vi "UpdateCaliperToCoorResultTable.vi"(7 "Type":enum16{"TagName", "Value"}(ring), 8 "error in (no error)":errorcluster, 10 "ProjectName":string, 11 "MCListbox Refnum":refnum<vi>) -> (0 "error out":errorcluster, 3 "CaliperResultNames":string[](array[string]))   [LabVIEW 2019]
uses:
  Controls/Caliper_Entry_FGV_Action.ctl
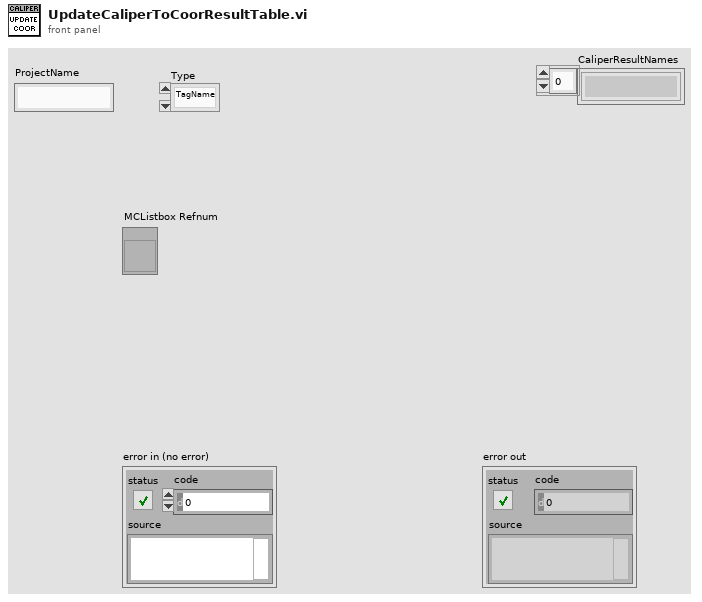
[diagram p1: front panel]
types:
  T1 = typedef "Caliper_Entry_FGV_Action.ctl" = enum16{"Init", "Close", "Add", "Delete", "ReplaceAll", "ReadAll"}
  T2 = typedef "CaliperDataEntry.ctl" = cluster{"CaliperType":T3, "Points":T4[], "Result":T6, "StepName":string}
  T3 = typedef "CaliperType.ctl" = u32
  T4 = typedef "SelectionListEntry.ctl" = cluster{"Type":T5, "Index":i32}
  T5 = typedef "SelectionListEntryPointType.ctl" = enum16{"AnalysisResult", "CaliperResult"}
  T6 = typedef "CaliperResult.ctl" = cluster{"PointInclude?":bool, "Num_Of_Pts":u8, "Position.X":dbl, "Position.Y":dbl, "Angle":dbl, "Distance":dbl, "Area":dbl, "Radius_MAX":dbl, "Radius2_min":dbl, "Dev_Residual":dbl, "P2.X":dbl, "P2.Y":dbl, "StepName":string, "Point ID":u8, "StepError?":bool, "ResultDiff?":bool}
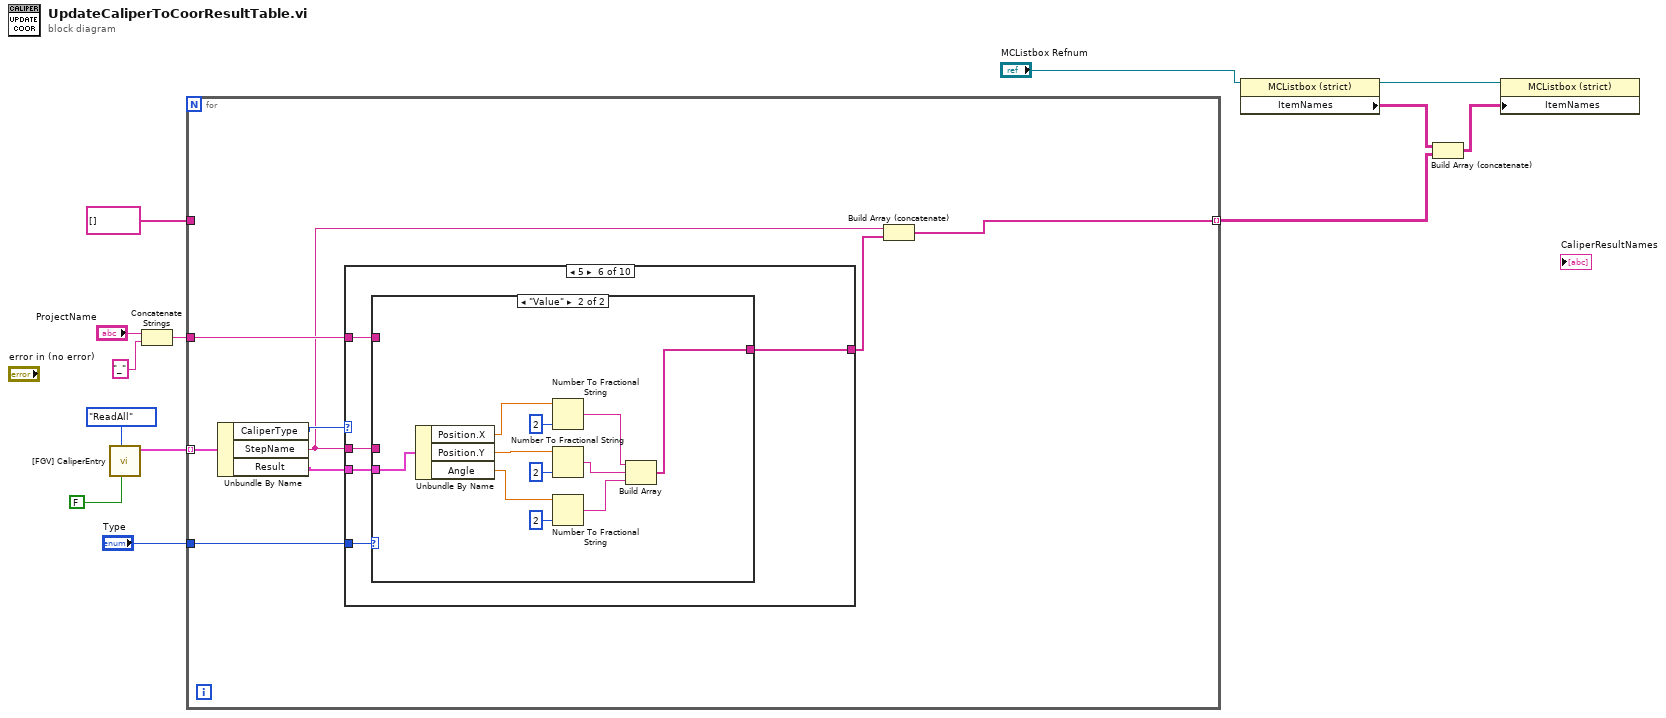
[diagram p0: block diagram]
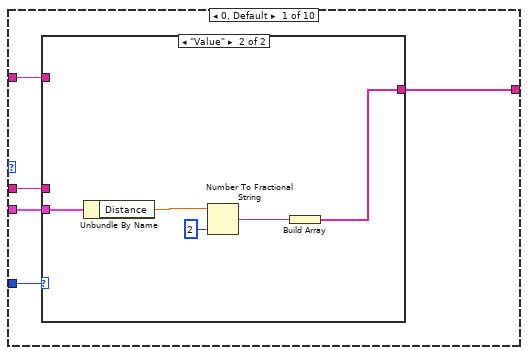
[diagram p2: hidden frame]
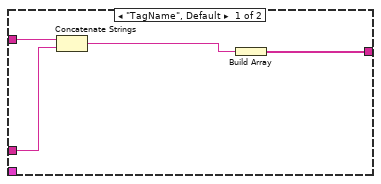
[diagram p3: hidden frame]
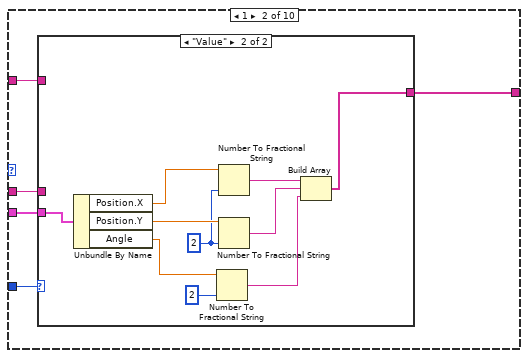
[diagram p4: hidden frame]
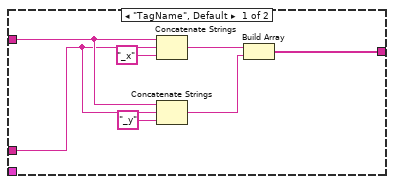
[diagram p5: hidden frame]
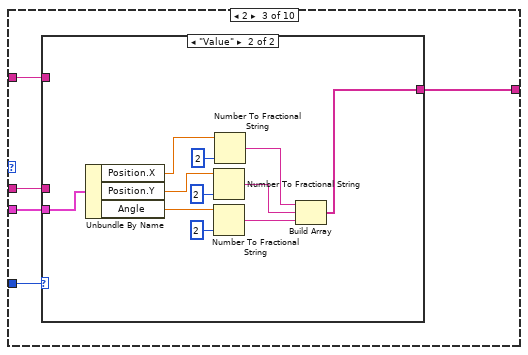
[diagram p6: hidden frame]
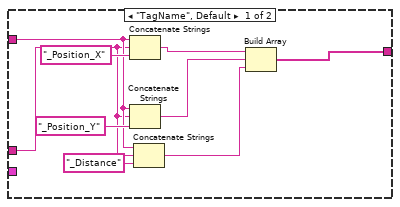
[diagram p7: hidden frame]
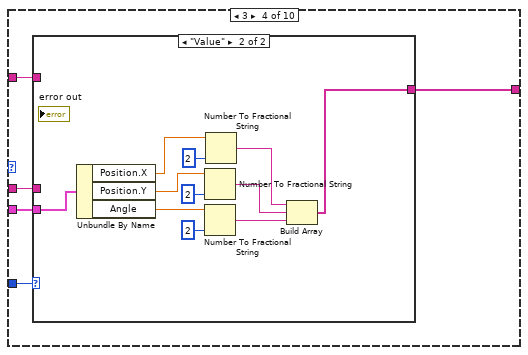
[diagram p8: hidden frame]
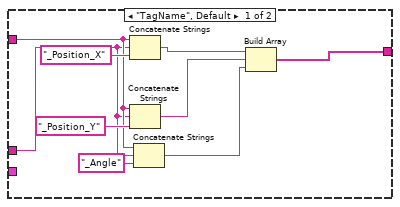
[diagram p9: hidden frame]
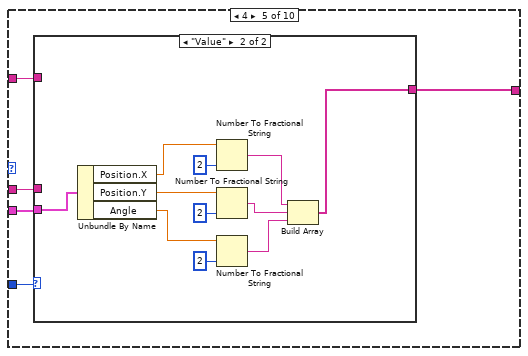
[diagram p10: hidden frame]
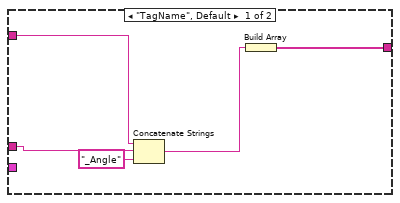
[diagram p11: hidden frame]
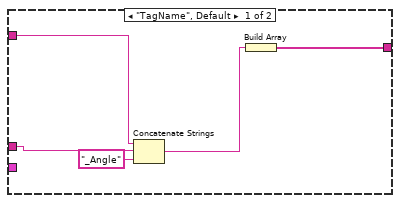
[diagram p12: hidden frame]
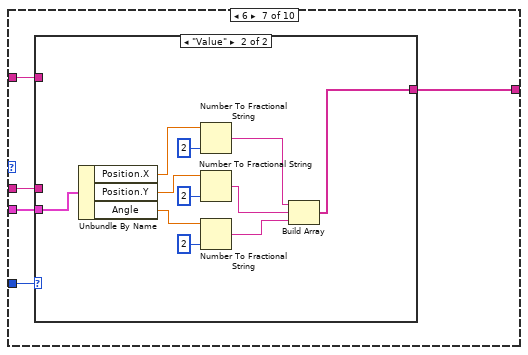
[diagram p13: hidden frame]
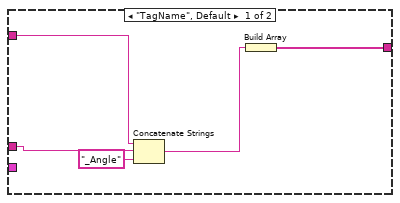
[diagram p14: hidden frame]
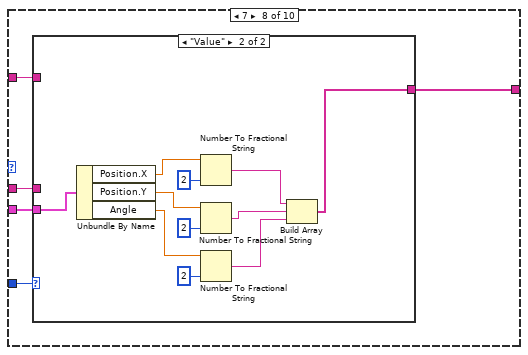
[diagram p15: hidden frame]
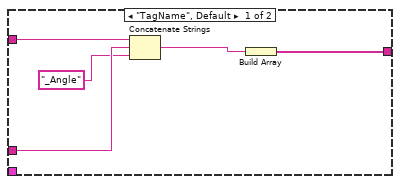
[diagram p16: hidden frame]
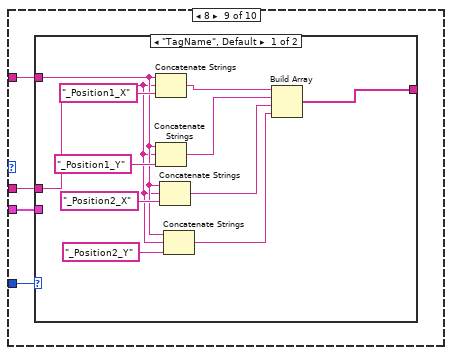
[diagram p17: hidden frame]
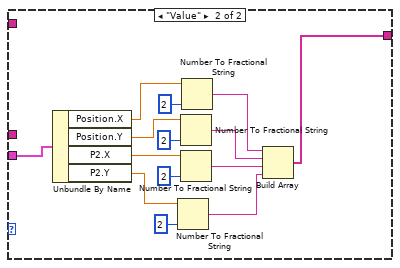
[diagram p18: hidden frame]
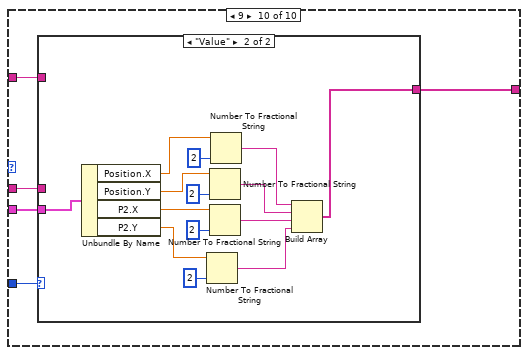
[diagram p19: hidden frame]
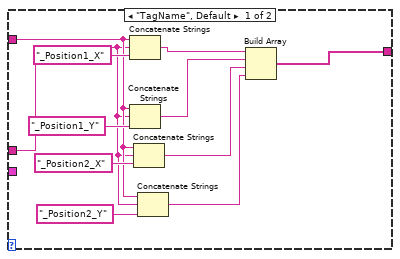
[diagram p20: hidden frame]
diagram:
  n1 = call "[FGV] CaliperEntry.vi"("CoordSystemRun"=FALSE, "Action"=Caliper_Entry_FGV_Action."ReadAll") -> ("AllCaliperEntries"=w12:T2[])  [unwired: 8 in, 1 out]
  n2 = Concatenate Strings("ProjectName", "_" ("string")) -> (w9:string)
  n3 = for {
    tunnel: w12 -> [w21] mode=indexing
    tunnel: w9 -> [w18]
    tunnel: "Type" -> [w17]
    tunnel: string[] [] -> [_]
    tunnel: [w14] -> w1 mode=indexing
    n4 = Unbundle By Name(w21) -> ("CaliperType"=w20:T3, "StepName"=w15:string, "Result"=w19:T6)
    n5 = case shown="5" w20 {
      tunnel: w15 -> [w25 w39 w59 w86 w109 w132 w153 w174 w194 w223]
      tunnel: w19 -> [w22 w36 w60 w83 w110 w131 w152 w171 w193 w222]
      tunnel: w18 -> [w26 w40 w61 w87 w111 w133 w154 w175 w195 w224]
      tunnel: [w24 w38 w62 w85 w112 w129 w151 w173 _ w225] -> w16
      tunnel: w17 -> [w23 w37 w58 w84 w108 w130 w150 w172 w192 w221]
      frame 0, Default {
        n6 = case shown="\"Value\"" w23 {
          tunnel: w26 -> [w30 _]
          tunnel: w25 -> [w29 _]
          tunnel: [w27 w31] -> w24
          tunnel: w22 -> [_ w35]
          frame "TagName", Default {
            n7 = Concatenate Strings(w30, w29) -> (w28:string)
            n8 = Build Array(w28) -> (w27:string[])
          }
          frame "Value" {
            n9 = Unbundle By Name(w35) -> ("Distance"=w34:dbl)
            n10 = Number To Fractional String(number=w34, precision (6)=i16 2) -> (F-format string=w32:string)  [unwired: 2 in]
            n11 = Build Array(w32) -> (w31:string[])
          }
        }
      }
      frame 1 {
        n12 = case shown="\"Value\"" w37 {
          tunnel: w40 -> [w47 _]
          tunnel: w39 -> [w46 _]
          tunnel: [w41 w52] -> w38
          tunnel: w36 -> [_ w57]
          frame "TagName", Default {
            n13 = Concatenate Strings(w47, w46, "_x" ("string")) -> (w43:string)
            n14 = Concatenate Strings(w47, w46, "_y" ("string")) -> (w42:string)
            n15 = Build Array(w43, w42) -> (w41:string[])
          }
          frame "Value" {
            w53 = i16 2 ("precision (6)")
            n16 = Unbundle By Name(w57) -> ("Position.X"=w55:dbl, "Position.Y"=w54:dbl, "Angle"=w50:dbl)
            n17 = Number To Fractional String(number=w50, precision (6)=i16 2) -> (F-format string=w49:string)  [unwired: 2 in]
            n18 = Number To Fractional String(number=w55, precision (6)=w53) -> (F-format string=w56:string)  [unwired: 2 in]
            n19 = Number To Fractional String(number=w54, precision (6)=w53) -> (F-format string=w48:string)  [unwired: 2 in]
            n20 = Build Array(w56, w48, w49) -> (w52:string[])
          }
        }
      }
      frame 2 {
        n21 = case shown="\"Value\"" w58 {
          tunnel: w61 -> [w66 _]
          tunnel: w59 -> [w65 _]
          tunnel: [w71 w78] -> w62
          tunnel: w60 -> [_ w79]
          frame "TagName", Default {
            n22 = Concatenate Strings(w66, w65, "_Position_X" ("string")) -> (w68:string)
            n23 = Concatenate Strings(w66, w65, "_Position_Y" ("string")) -> (w67:string)
            n24 = Concatenate Strings(w66, w65, "_Distance" ("string")) -> (w63:string)
            n25 = Build Array(w68, w67, w63) -> (w71:string[])
          }
          frame "Value" {
            n26 = Unbundle By Name(w79) -> ("Position.X"=w75:dbl, "Position.Y"=w74:dbl, "Angle"=w82:dbl)
            n27 = Number To Fractional String(number=w74, precision (6)=i16 2) -> (F-format string=w72:string)  [unwired: 2 in]
            n28 = Number To Fractional String(number=w82, precision (6)=i16 2) -> (F-format string=w80:string)  [unwired: 2 in]
            n29 = Number To Fractional String(number=w75, precision (6)=i16 2) -> (F-format string=w73:string)  [unwired: 2 in]
            n30 = Build Array(w73, w72, w80) -> (w78:string[])
          }
        }
      }
      frame 3 {
        n31 = case shown="\"Value\"" w84 {
          tunnel: w87 -> [w91 _]
          tunnel: w86 -> [w90 _]
          tunnel: [w96 w103] -> w85
          tunnel: w83 -> [_ w104]
          frame "TagName", Default {
            n32 = Concatenate Strings(w91, w90, "_Position_X" ("string")) -> (w93:string)
            n33 = Concatenate Strings(w91, w90, "_Position_Y" ("string")) -> (w92:string)
            n34 = Concatenate Strings(w91, w90, "_Angle" ("string")) -> (w88:string)
            n35 = Build Array(w93, w92, w88) -> (w96:string[])
          }
          frame "Value" {
            n36 = Unbundle By Name(w104) -> ("Position.X"=w100:dbl, "Position.Y"=w99:dbl, "Angle"=w107:dbl)
            n37 = Number To Fractional String(number=w99, precision (6)=i16 2) -> (F-format string=w97:string)  [unwired: 2 in]
            n38 = Number To Fractional String(number=w107, precision (6)=i16 2) -> (F-format string=w105:string)  [unwired: 2 in]
            n39 = Number To Fractional String(number=w100, precision (6)=i16 2) -> (F-format string=w98:string)  [unwired: 2 in]
            n40 = Build Array(w98, w97, w105) -> (w103:string[])
          }
        }
      }
      frame 4 {
        n41 = case shown="\"Value\"" w108 {
          tunnel: w111 -> [w114 _]
          tunnel: w109 -> [w113 _]
          tunnel: [w117 w124] -> w112
          tunnel: w110 -> [_ w125]
          frame "TagName", Default {
            n42 = Concatenate Strings(w114, w113, "_Angle" ("string")) -> (w115:string)
            n43 = Build Array(w115) -> (w117:string[])
          }
          frame "Value" {
            n44 = Unbundle By Name(w125) -> ("Position.X"=w121:dbl, "Position.Y"=w120:dbl, "Angle"=w128:dbl)
            n45 = Number To Fractional String(number=w121, precision (6)=i16 2) -> (F-format string=w118:string)  [unwired: 2 in]
            n46 = Number To Fractional String(number=w120, precision (6)=i16 2) -> (F-format string=w119:string)  [unwired: 2 in]
            n47 = Number To Fractional String(number=w128, precision (6)=i16 2) -> (F-format string=w126:string)  [unwired: 2 in]
            n48 = Build Array(w118, w119, w126) -> (w124:string[])
          }
        }
      }
      frame 5 {
        n49 = case shown="\"Value\"" w130 {
          tunnel: w133 -> [w135 _]
          tunnel: w132 -> [w134 _]
          tunnel: [w138 w145] -> w129
          tunnel: w131 -> [_ w146]
          frame "TagName", Default {
            n50 = Concatenate Strings(w135, w134, "_Angle" ("string")) -> (w136:string)
            n51 = Build Array(w136) -> (w138:string[])
          }
          frame "Value" {
            n52 = Unbundle By Name(w146) -> ("Position.X"=w140:dbl, "Position.Y"=w143:dbl, "Angle"=w149:dbl)
            n53 = Number To Fractional String(number=w140, precision (6)=i16 2) -> (F-format string=w139:string)  [unwired: 2 in]
            n54 = Number To Fractional String(number=w143, precision (6)=i16 2) -> (F-format string=w142:string)  [unwired: 2 in]
            n55 = Number To Fractional String(number=w149, precision (6)=i16 2) -> (F-format string=w147:string)  [unwired: 2 in]
            n56 = Build Array(w139, w142, w147) -> (w145:string[])
          }
        }
      }
      frame 6 {
        n57 = case shown="\"Value\"" w150 {
          tunnel: w154 -> [w156 _]
          tunnel: w153 -> [w155 _]
          tunnel: [w159 w166] -> w151
          tunnel: w152 -> [_ w167]
          frame "TagName", Default {
            n58 = Concatenate Strings(w156, w155, "_Angle" ("string")) -> (w157:string)
            n59 = Build Array(w157) -> (w159:string[])
          }
          frame "Value" {
            n60 = Unbundle By Name(w167) -> ("Position.X"=w163:dbl, "Position.Y"=w162:dbl, "Angle"=w170:dbl)
            n61 = Number To Fractional String(number=w163, precision (6)=i16 2) -> (F-format string=w161:string)  [unwired: 2 in]
            n62 = Number To Fractional String(number=w162, precision (6)=i16 2) -> (F-format string=w160:string)  [unwired: 2 in]
            n63 = Number To Fractional String(number=w170, precision (6)=i16 2) -> (F-format string=w168:string)  [unwired: 2 in]
            n64 = Build Array(w161, w160, w168) -> (w166:string[])
          }
        }
      }
      frame 7 {
        n65 = case shown="\"Value\"" w172 {
          tunnel: w175 -> [w180 _]
          tunnel: w174 -> [w179 _]
          tunnel: [w177 w187] -> w173
          tunnel: w171 -> [_ w188]
          frame "TagName", Default {
            n66 = Concatenate Strings(w180, w179, "_Angle" ("string")) -> (w178:string)
            n67 = Build Array(w178) -> (w177:string[])
          }
          frame "Value" {
            n68 = Unbundle By Name(w188) -> ("Position.X"=w183:dbl, "Position.Y"=w184:dbl, "Angle"=w191:dbl)
            n69 = Number To Fractional String(number=w183, precision (6)=i16 2) -> (F-format string=w181:string)  [unwired: 2 in]
            n70 = Number To Fractional String(number=w184, precision (6)=i16 2) -> (F-format string=w182:string)  [unwired: 2 in]
            n71 = Number To Fractional String(number=w191, precision (6)=i16 2) -> (F-format string=w189:string)  [unwired: 2 in]
            n72 = Build Array(w181, w182, w189) -> (w187:string[])
          }
        }
      }
      frame 8 {
        n73 = case shown="\"TagName\", Default" w192 {
          tunnel: w195 -> [w197 _]
          tunnel: w194 -> [w196 _]
          tunnel: [w206 w217] -> _
          tunnel: w193 -> [_ w218]
          frame "TagName", Default {
            n74 = Concatenate Strings(w197, w196, "_Position1_X" ("string")) -> (w203:string)
            n75 = Concatenate Strings(w197, w196, "_Position1_Y" ("string")) -> (w202:string)
            n76 = Concatenate Strings(w197, w196, "_Position2_X" ("string")) -> (w200:string)
            n77 = Concatenate Strings(w197, w196, "_Position2_Y" ("string")) -> (w198:string)
            n78 = Build Array(w203, w202, w200, w198) -> (w206:string[])
          }
          frame "Value" {
            n79 = Unbundle By Name(w218) -> ("Position.X"=w214:dbl, "Position.Y"=w213:dbl, "P2.X"=w220:dbl, "P2.Y"=w208:dbl)
            n80 = Number To Fractional String(number=w208, precision (6)=i16 2) -> (F-format string=w207:string)  [unwired: 2 in]
            n81 = Number To Fractional String(number=w213, precision (6)=i16 2) -> (F-format string=w211:string)  [unwired: 2 in]
            n82 = Number To Fractional String(number=w220, precision (6)=i16 2) -> (F-format string=w219:string)  [unwired: 2 in]
            n83 = Number To Fractional String(number=w214, precision (6)=i16 2) -> (F-format string=w212:string)  [unwired: 2 in]
            n84 = Build Array(w212, w211, w219, w207) -> (w217:string[])
          }
        }
      }
      frame 9 {
        n85 = case shown="\"Value\"" w221 {
          tunnel: w224 -> [w227 _]
          tunnel: w223 -> [w226 _]
          tunnel: [w236 w247] -> w225
          tunnel: w222 -> [_ w248]
          frame "TagName", Default {
            n86 = Concatenate Strings(w227, w226, "_Position1_X" ("string")) -> (w233:string)
            n87 = Concatenate Strings(w227, w226, "_Position1_Y" ("string")) -> (w232:string)
            n88 = Concatenate Strings(w227, w226, "_Position2_X" ("string")) -> (w230:string)
            n89 = Concatenate Strings(w227, w226, "_Position2_Y" ("string")) -> (w228:string)
            n90 = Build Array(w233, w232, w230, w228) -> (w236:string[])
          }
          frame "Value" {
            n91 = Unbundle By Name(w248) -> ("Position.X"=w244:dbl, "Position.Y"=w243:dbl, "P2.X"=w250:dbl, "P2.Y"=w238:dbl)
            n92 = Number To Fractional String(number=w238, precision (6)=i16 2) -> (F-format string=w237:string)  [unwired: 2 in]
            n93 = Number To Fractional String(number=w243, precision (6)=i16 2) -> (F-format string=w241:string)  [unwired: 2 in]
            n94 = Number To Fractional String(number=w250, precision (6)=i16 2) -> (F-format string=w249:string)  [unwired: 2 in]
            n95 = Number To Fractional String(number=w244, precision (6)=i16 2) -> (F-format string=w242:string)  [unwired: 2 in]
            n96 = Build Array(w242, w241, w249, w237) -> (w247:string[])
          }
        }
      }
    }
    n97 = Build Array (concatenate)(w15, w16) -> (w14:string[])
  }
  n98 = property class="MCListbox (strict)"(reference="MCListbox Refnum") -> (reference out=w3:refnum<vi>, "ItemNames"=w5:string[][])  [unwired: 1 in, 1 out]
  n99 = Build Array (concatenate)(w5, w1) -> (w4:string[][])
  n100 = property class="MCListbox (strict)"(reference=w3, "ItemNames"=w4) -> ()  [unwired: 1 in, 2 out]
